vi "Create Slice String.vi"(7 "3D Pie Property":T5, 8 "error in (no error)":errorcluster, 9 "Actual Transform In":T1, 10 "Plot Representation In":T3, 11 "Plot Object In":refnum<vi>) -> (0 "error out":errorcluster, 1 "Actual Transform Out":T1, 2 "Plot Representation Out":T3, 3 "Plot Object Out":refnum<vi>)   [LabVIEW 2017, in "3D Pie.lvclass"]
uses:
  <vilib>/Math Plots/3D Math Plots/3D Pie/3D Pie/3D Pie.lvclass
  <vilib>/Math Plots/3D Math Plots/3D Pie/3D Pie/Typedef/3D Pie Property.ctl
  <vilib>/Math Plots/3D Math Plots/3D Plot/3D Plot/Typedef/Line Type.ctl
  <vilib>/Math Plots/3D Math Plots/3D Plot/3D Plot/Typedef/Plot Representation.ctl
  <vilib>/Math Plots/3D Math Plots/3D Plot/3D Plot/Typedef/Range Clusters.ctl
  <vilib>/Math Plots/3D Math Plots/3D Plot/3D Plot/Typedef/Mesh Data.ctl
  <vilib>/Math Plots/3D Math Plots/3D Plot/3D Plot/Typedef/Actual Transform.ctl
  <vilib>/Math Plots/3D Math Plots/3D Plot/3D Plot/3D Plot.lvclass
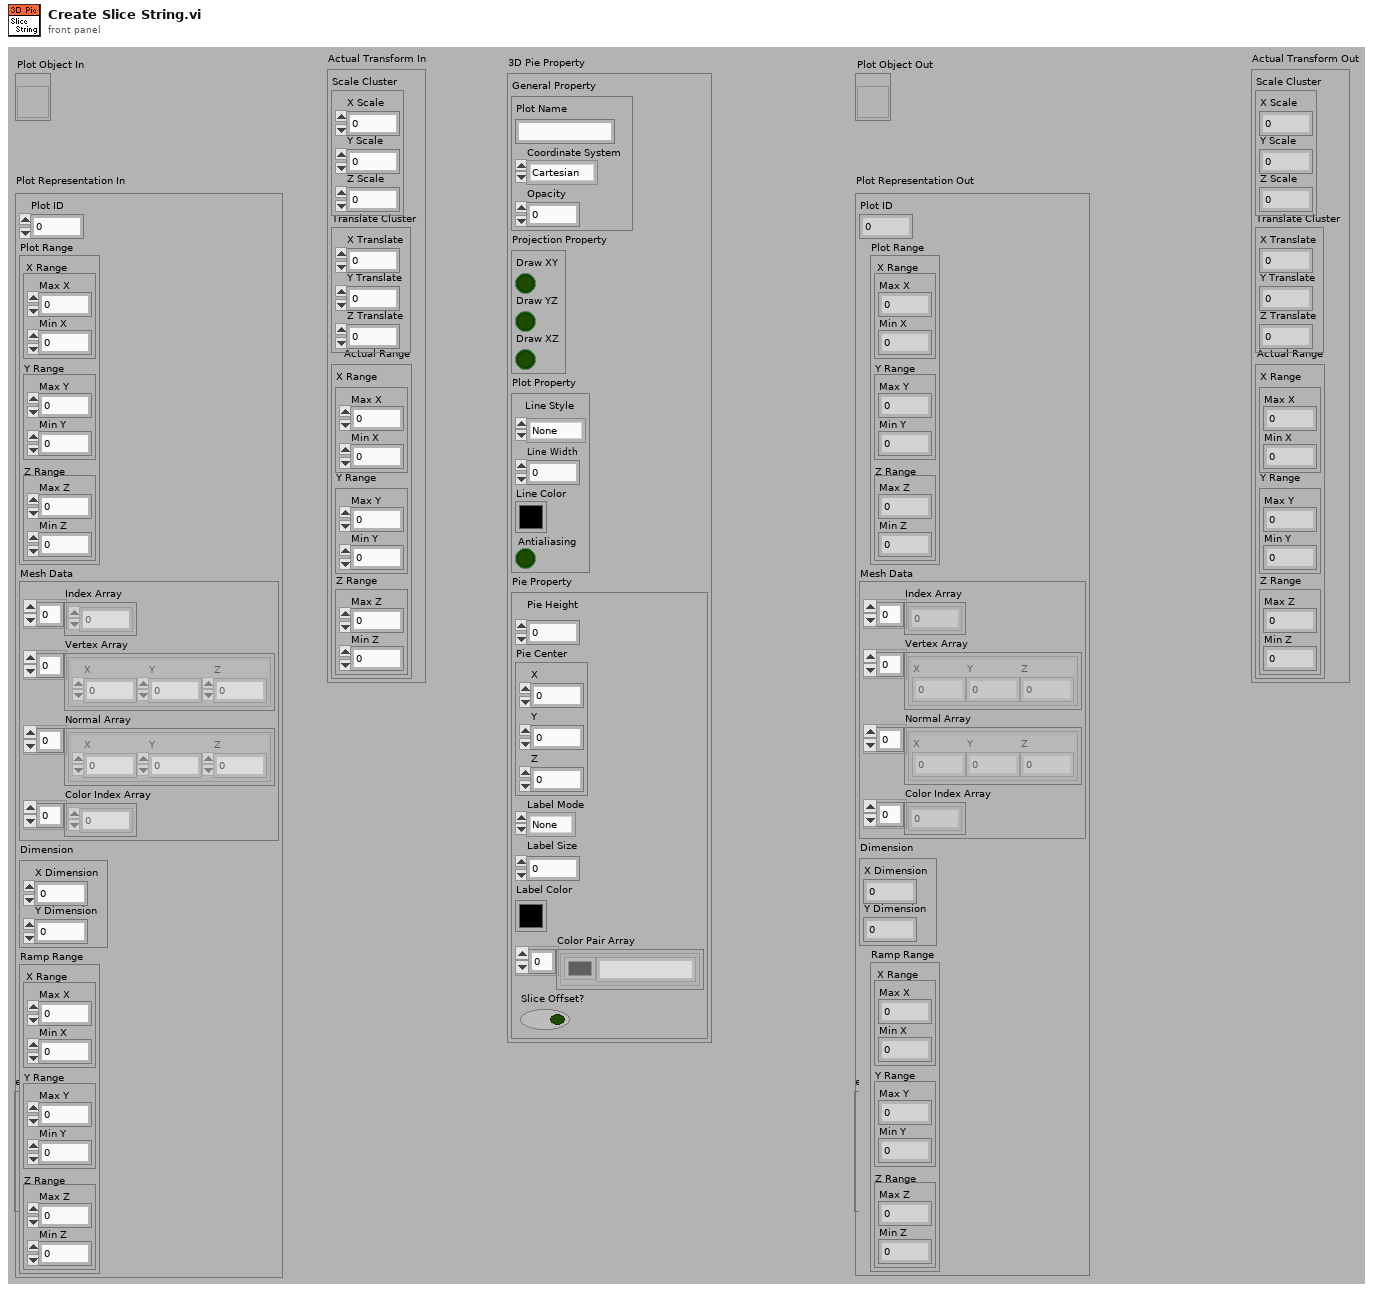
[diagram p1: front panel]
types:
  T1 = typedef "3D Plot.lvclass/Actual Transform.ctl" = cluster{"Scale Cluster":cluster{"X Scale":sgl, "Y Scale":sgl, "Z Scale":sgl}, "Translate Cluster":cluster{"X Translate":sgl, "Y Translate":sgl, "Z Translate":sgl}, "Actual Range":T2}
  T2 = typedef "3D Plot.lvclass/Range Clusters.ctl" = cluster{"X Range":cluster{"Max X":sgl, "Min X":sgl}, "Y Range":cluster{"Max Y":sgl, "Min Y":sgl}, "Z Range":cluster{"Max Z":sgl, "Min Z":sgl}}
  T3 = typedef "3D Plot.lvclass/Plot Representation.ctl" = cluster{"Plot ID":i32, "Plot Range":T2, "Mesh Data":T4, "Dimension":cluster{"X Dimension":i32, "Y Dimension":i32}, "Ramp Range":T2}
  T4 = typedef "3D Plot.lvclass/Mesh Data.ctl" = cluster{"Index Array":u32[], "Vertex Array":cluster{"X":sgl, "Y":sgl, "Z":sgl}[], "Normal Array":cluster{"X":sgl, "Y":sgl, "Z":sgl}[], "Color Index Array":i32[]}
  T5 = typedef "3D Pie.lvclass/3D Pie Property.ctl" = cluster{"General Property":cluster{"Plot Name":string, "Coordinate System":enum16{"Cartesian", "Cylindrical", "Spherical"}, "Opacity":sgl}, "Projection Property":cluster{"Draw XY":bool, "Draw YZ":bool, "Draw XZ":bool}, "Plot Property":cluster{"Line Style":T6, "Line Width":sgl, "Line Color":u32, "Antialiasing":bool}, "Pie Property":cluster{"Pie Height":sgl, "Pie Center":cluster{"X":sgl, "Y":sgl, "Z":sgl}, "Label Mode":enum16{"None", "Show Percentage", "Show String"}, "Label Size":u16, "Label Color":u32, "Color Pair Array":cluster{"Color":u32, "String":string}[], "Slice Offset?":bool}}
  T6 = typedef "3D Plot.lvclass/Line Type.ctl" = enum16{"None", "Solid", "Dash", "Dot", "Dash Dot"}
  T7 = enum16{"Normal Bin", "Opaque Bin", "Transparent Bin"}
  T8 = cluster{"X Scale":sgl, "Y Scale":sgl, "Z Scale":sgl}
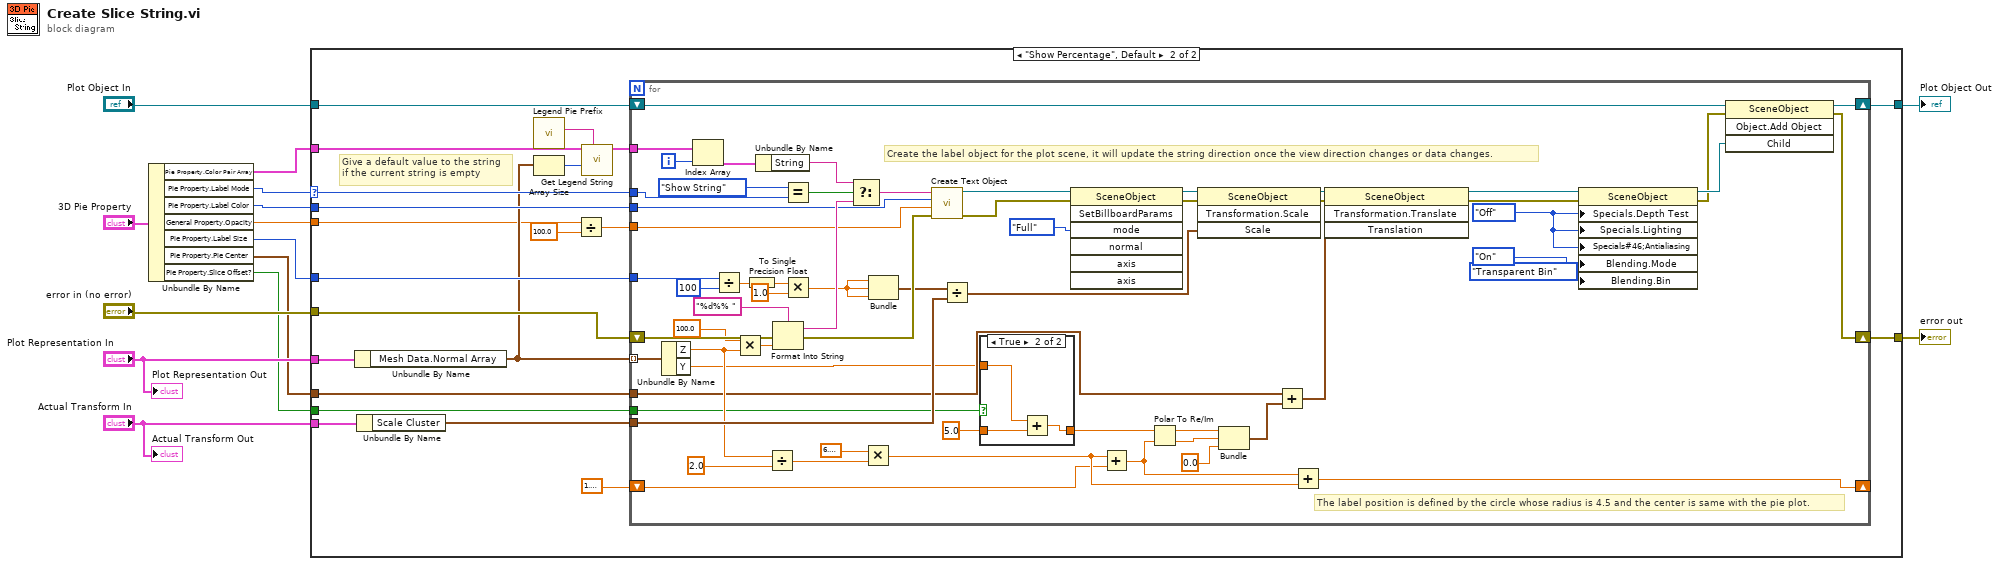
[diagram p0: block diagram]
diagram:
  n1 = Unbundle By Name("3D Pie Property") -> ("Pie Property.Color Pair Array"=w6:cluster{"Color":u32, "String":string}[], "Pie Property.Label Mode"=w13:enum16{"None", "Show Percentage", "Show String"}, "Pie Property.Label Color"=w11:u32, "General Property.Opacity"=w5:sgl, "Pie Property.Label Size"=w8:u16, "Pie Property.Pie Center"=w2:cluster{"X":sgl, "Y":sgl, "Z":sgl}, "Pie Property.Slice Offset?"=w1:bool)
  n2 = case shown="\"Show Percentage\", Default" w13 {
    selector: w13 -> [_ w37]
    tunnel: "Plot Representation In" -> [_ w20]
    tunnel: w6 -> [_ w28]
    tunnel: "error in (no error)" -> [w15 w36]
    tunnel: w11 -> [_ w35]
    tunnel: "Plot Object In" -> [w16 w34]
    tunnel: [w16 w33] -> w9
    tunnel: "Actual Transform In" -> [_ w29]
    tunnel: w8 -> [_ w32]
    tunnel: [w15 w30] -> w7
    tunnel: w5 -> [_ w23]
    tunnel: w2 -> [_ w18]
    tunnel: w1 -> [_ w17]
    frame "None" {
    }
    frame "Show Percentage", Default {
      # "Give a default value to the string\nif the current string is empty"
      n3 = Unbundle By Name(w20) -> ("Mesh Data.Normal Array"=w27:cluster{"X":sgl, "Y":sgl, "Z":sgl}[])
      n4 = Unbundle By Name(w29) -> ("Scale Cluster"=w21:T8)
      n5 = call <vilib>:"Legend Pie Prefix.vi"() -> ("Prefix Out"=w19:string)  [unwired: 11 out]
      n6 = Array Size(array=w27) -> (size(s)=w25:i32)
      n7 = Divide(x=w23, y=sgl 100.0) -> (x/y=w22:sgl)
      n8 = call <vilib>:"Get Legend String.vi"("Initial String"=w19, "Pair Array Length"=w25, "Color Pair Array In"=w28) -> ("Color Pair Array Out"=w26:cluster{"Color":u32, "String":string}[])  [unwired: 2 in, 6 out]
      n9 = for {
        tunnel: w27 -> [w98] mode=indexing
        tunnel: w37 -> [w97]
        tunnel: w35 -> [w52]
        shift-right: [w80] -> w33
        shift-left: w34 -> [w81]
        tunnel: w32 -> [w73]
        tunnel: w21 -> [w72]
        shift-right: [w62] -> _
        shift-left: sgl 1.5707964 -> [w63]
        shift-right: [w60] -> w30
        shift-left: w36 -> [w90]
        tunnel: w26 -> [w55]
        tunnel: w22 -> [w51]
        tunnel: w18 -> [w41]
        tunnel: w17 -> [w40]
        i -> [w56]
        w45 = enum16{"Inherit Value", "Off", "On"}."Off" ("Specials:Lighting")
        # "The label position is defined by the circle whose radius is 4.5 and the center is same with the pie plot."
        # "Create the label object for the plot scene, it will update the string direction once the view direction changes or data changes."
        n10 = Unbundle By Name(w98) -> ("Z"=w59:sgl, "Y"=w38:sgl)
        n11 = Index Array(array=w55, index=w56) -> (element=w54:cluster{"Color":u32, "String":string})
        n12 = Divide(x=w73, y=100) -> (x/y=w78:dbl)
        n13 = Multiply(x=sgl 100.0, y=w59) -> (x*y=w57:sgl)
        n14 = To Single Precision Float(number=w78) -> (single precision float=w44:sgl)
        n15 = Unbundle By Name(w54) -> ("String"=w53:string)
        n16 = Divide(x=w59, y=sgl 2.0) -> (x/y=w66:sgl)
        n17 = Format Into String(format string="%d%% ", error in=w90, w57) -> (resulting string=w93:string, error out=w91:errorcluster)  [unwired: 1 in]
        n18 = Equal?(x=enum16{"None", "Show Percentage", "Show String"}."Show String" ("Label Mode"), y=w97) -> (x = y?=w95:bool)
        n19 = Multiply(x=w44, y=sgl 1.0 ("Length")) -> (x*y=w77:sgl)
        n20 = Select(t=w53, s=w95, f=w93) -> (s? t:f=w92:string)
        n21 = Multiply(x=sgl 6.2831855, y=w66) -> (x*y=w64:sgl)
        n22 = Bundle(w77, w77, w77) -> (w76:cluster{sgl, sgl, sgl})  [unwired: 1 out]
        n23 = call <vilib>:"Create Text Object.vi"("error in (no error)"=w91, "Alpha"=w51, "Color Box"=w52, "Value String"=w92) -> ("error out"=w48:errorcluster, "Scene:New Object"=w49:refnum<vi>)  [unwired: 6 out]
        n24 = Divide(x=w76, y=w72) -> (x/y=w74:cluster{sgl, sgl, sgl})
        n25 = case shown="True" w40 {
          tunnel: [w99 w101] -> w61
          tunnel: sgl 5.0 ("r") -> [w99 w102]
          tunnel: w38 -> [_ w100]
          frame False {
          }
          frame True {
            n26 = Add(x=w100, y=w102) -> (x+y=w101:sgl)
          }
        }
        n27 = invoke class="SceneObject" method="SetBillboardParams"(reference=w49, error in=w48, "mode"=enum16{"No Billboarding", "Axial", "Full"}."Full") -> (reference out=w47:refnum<vi>, error out=w46:errorcluster)  [unwired: 4 in, 5 out]
        n28 = Add(x=w64, y=w63) -> (x+y=w65:sgl)
        n29 = Polar To Re/Im(2:w65, 3:w61) -> (0:w67:sgl, 1:w68:sgl)
        n30 = invoke class="SceneObject" method="Transformation.Scale"(reference=w47, error in=w46, "Scale"=w74) -> (reference out=w89:refnum<vi>, error out=w88:errorcluster)  [unwired: 1 in, 2 out]
        n31 = Bundle(w68, w67, "y"=sgl 0.0) -> (w43:cluster{sgl, sgl, "y":sgl})  [unwired: 1 out]
        n32 = Add(x=w41, y=w43) -> (x+y=w42:cluster{sgl, sgl, sgl})
        n33 = Add(x=w65, y=w64) -> (x+y=w62:sgl)
        n34 = invoke class="SceneObject" method="Transformation.Translate"(reference=w89, error in=w88, "Translation"=w42) -> (reference out=w84:refnum<vi>, error out=w85:errorcluster)  [unwired: 1 in, 2 out]
        n35 = property class="SceneObject"(reference=w84, error in=w85, "Specials.Depth Test"=w45, "Specials.Lighting"=w45, "Specials#46;Antialiasing"=w45, "Blending.Mode"=enum16{"Inherit Value", "Off", "On"}."On" ("Blending:Mode"), "Blending.Bin"=T7."Transparent Bin" ("Blending:Bin")) -> (reference out=w83:refnum<vi>, error out=w82:errorcluster)
        n36 = invoke class="SceneObject" method="Object.Add Object"(reference=w81, error in=w82, "Child"=w83) -> (reference out=w80:refnum<vi>, error out=w60:errorcluster)  [unwired: 1 in, 2 out]
      }
    }
  }
  "Plot Object Out" <- w9
  "error out" <- w7
  "Plot Representation Out" <- "Plot Representation In"
  "Actual Transform Out" <- "Actual Transform In"
